vi "RegisterDataSetsRoutedMessage_Name.vi"() -> (1 "message name":string="McsaDataEventCreator.RegisterDataSet")   [LabVIEW 2017, in "McsaDataEventCreator.lvlib"]
uses:
  <vilib>/addons/InsightCM/Devices/Shared/Mcsa/McsaDataEventCreator/McsaDataEventCreator.lvlib
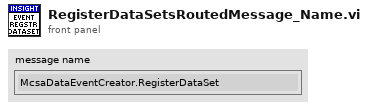
[diagram p1: front panel]
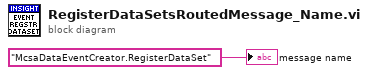
[diagram p0: block diagram]
diagram:
  "message name" <- "McsaDataEventCreator.RegisterDataSet" ("ProcessName")
